vi "Configure Network Subnet Mask.vi"(8 "error in (no error)":errorcluster, 10 "Subnet Mask (\"\")":string, 11 "VISA resource name":refnum<visa-resource-name>) -> (0 "error out":errorcluster, 3 "VISA resource name out":refnum<visa-resource-name>)   [LabVIEW 2015, in "Rohde&Schwarz CMXP Base.lvlib"]
doc: "Manually defines the subnet masks to be used for the network adapter IPv4 addresses. A query returns the currently used subnet masks, irrespective of whether they have been assigned manually or via DHCP.\n\nAttribute:\nRSCMXPBASE_ATTR_CONFIGURE_NETWORK_SUBNET_MASK\n\nRemote-control command:\nSYSTem:COMMunicate:NET:SUBNet:MASK"
uses:
  <instrlib>/Rohde&Schwarz CMXP Base/Rohde&Schwarz CMXP Base.lvlib
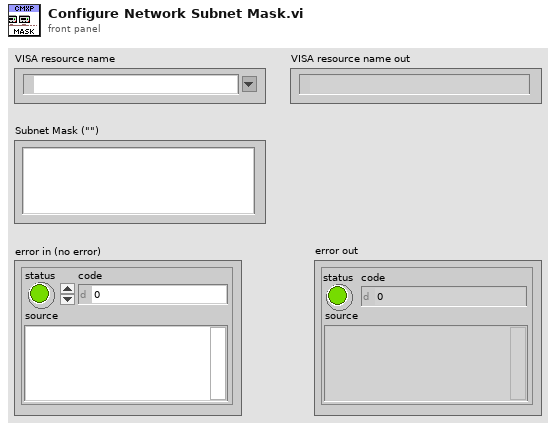
[diagram p1: front panel]
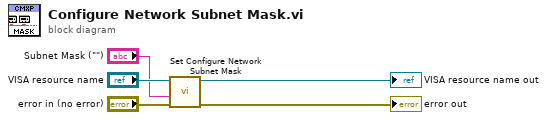
[diagram p0: block diagram]
diagram:
  n1 = call "Set Configure Network Subnet Mask"("error in (no error)"="error in (no error)", "Configure Network Subnet Mask ()"="Subnet Mask (\"\")", "instrument handle"="VISA resource name") -> ("error out"=→"error out":errorcluster, "instrument handle out"=→"VISA resource name out":refnum<visa-resource-name>)  [unwired: 7 in]
